vi "FFT Test.vi"() -> ()   [LabVIEW 2012, in "OpenCLV x64.lvlib"]
uses:
  OpenCLV x64.lvlib
  <vilib>/Analysis/2dsp.llb/2D Real FFT.vi
  <vilib>/Analysis/2dsp.llb/2D Inverse Real FFT.vi
  <vilib>/Analysis/2dsp.llb/Real FFT.vi
  <vilib>/Analysis/NI_AALPro.lvlib
panel:
  out "X":dbl[][](array[numeric])
  out "FFT {X}":cdb[][](array[numeric])
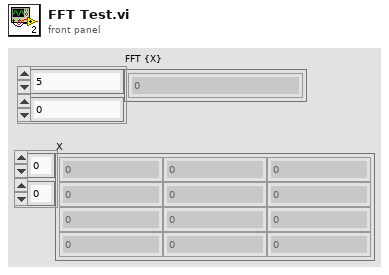
[diagram p1: front panel]
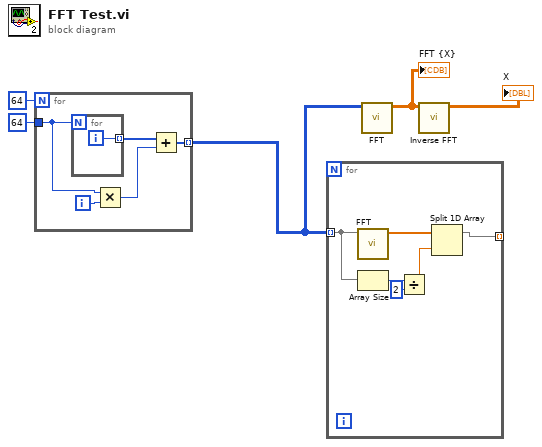
[diagram p0: block diagram]
diagram:
  n1 = for {
    N: 64 -> [_]
    tunnel: 64 -> [w8]
    tunnel: [w6] -> w3 mode=indexing
    i -> [w9]
    n2 = for {
      N: w8 -> [_]
      tunnel: [w11] -> w10 mode=indexing
      i -> [w11]
    }
    n3 = Multiply(x=w8, y=w9) -> (x*y=w7:i32)
    n4 = Add(x=w10, y=w7) -> (x+y=w6:i32[])
  }
  n5 = for {
    tunnel: w3 -> [w17] mode=indexing
    tunnel: [w12] -> _ mode=indexing
    n6 = call-poly <vilib>:"FFT.vi"("X"=w17) -> ("FFT {X}"=w14:cdb[])  [unwired: 9 in, 1 out]
    n7 = Array Size(array=w17) -> (size(s)=w16:i32)
    n8 = Divide(x=w16, y=2) -> (x/y=w13:dbl)
    n9 = Split 1D Array(array=w14, index=w13) -> (first subarray=w12:cdb[])  [unwired: 1 out]
  }
  n10 = call-poly <vilib>:"FFT.vi"("X"=w3) -> ("FFT {X}"=w2:cdb[][])  [unwired: 9 in, 1 out]
  "FFT {X}" <- w2
  n11 = call-poly <vilib>:"Inverse FFT.vi"("FFT {X}"=w2) -> ("X"=→"X":dbl[][])  [unwired: 9 in, 1 out]
